vi "Save Project.vi"(7 "index":i32, 8 "error in":errorcluster, 11 "Builder in":refnum<class "Builder.lvclass">) -> (0 "error out":errorcluster, 3 "Builder out":refnum<class "Builder.lvclass">)   [LabVIEW 2021, in "App-Builder Library.lvlib" / "Builder.lvclass"]
uses:
  Builder.lvclass
  Builder.lvclass/Builder.ctl
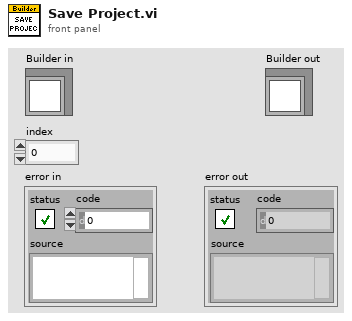
[diagram p1: front panel]
types:
  T1 = typedef "App-Builder Library.lvlib/Builder.lvclass/Build specification.ctl" = cluster{"target name":string, "Build specification":string, "Project Path":path, "Build Object type":T2}
  T2 = typedef "App-Builder Library.lvlib/Builder.lvclass/Build object type.ctl" = enum16{"Source Distribution", "Deployable Source Distribution", "DLL", "EXE", "Packed Library", "Deployable Packed", "RT EXE", ".NET Interop Assembly"}
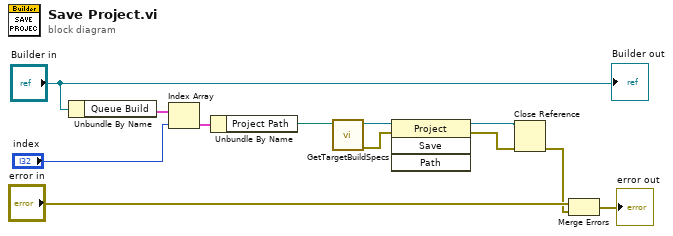
[diagram p0: block diagram]
diagram:
  n1 = Unbundle By Name("Builder in") -> ("Queue Build"=w4:T1[])
  n2 = Index Array(array=w4, index="index") -> (element=w2:T1)
  n3 = Unbundle By Name(w2) -> ("Project Path"=w1:path)
  n4 = call <vilib>:"GetTargetBuildSpecs.vi"("Path to project"=w1) -> ("error out"=w6:errorcluster, "project ref"=w10:refnum<vi>)  [unwired: 8 in, 1 out]
  n5 = invoke class="Project" method="Save"(reference=w10, error in=w6) -> (reference out=w9:refnum<vi>, error out=w8:errorcluster)  [unwired: 2 in, 2 out]
  n6 = Close Reference(reference=w9, error in (no error)=w8) -> (error out=w7:errorcluster)
  n7 = Merge Errors("error in", w7) -> (→"error out":errorcluster)
  "Builder out" <- "Builder in"
